vi "GT Get Soft Limit.vi"(7 "pNegative":i32, 8 "error in (no error)":errorcluster caption="错误输入（无错误）", 9 "pPositive":i32, 10 "axis":i16, 11 "cardNum":i16) -> (0 "error out":errorcluster caption="错误输出", 1 "pPositive out":i32, 3 "function return":i16, 5 "pNegative out":i32)   [LabVIEW 2014, in "gts.lvlib"]
doc: "GT_API GT_GetSoftLimit(short cardNum,short axis,long *pPositive,long *pNegative);"
uses:
  gts.lvlib
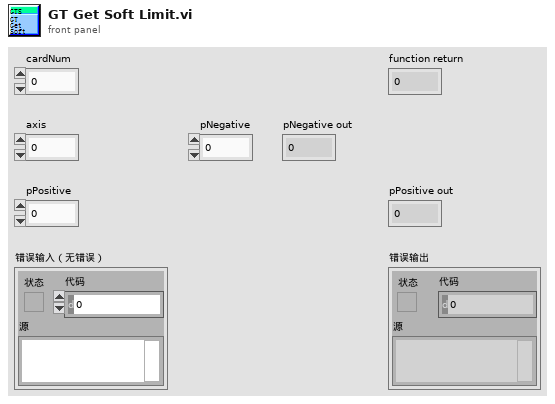
[diagram p1: front panel]
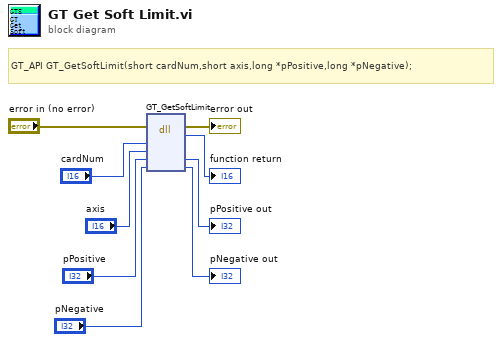
[diagram p0: block diagram]
diagram:
  # "GT_API GT_GetSoftLimit(short cardNum,short axis,long *pPositive,long *pNegative);"
  n1 = dll-call lib="PTH2habs D固高科技资料GTS控制卡GTS卡18年上半年资料dllVC32bit\nmulti_cardgts.*" fn="GT_GetSoftLimit"(error in="error in (no error)", "cardNum"="cardNum", "axis"="axis", "pPositive"="pPositive", "pNegative"="pNegative") -> (error out=→"error out":errorcluster, →"function return":i16, "pPositive"=→"pPositive out":i32, "pNegative"=→"pNegative out":i32)  [unwired: 4 in, 1 out]
